vi "InitialPulseDelta6221_ver2.0.vi"(1 "Keithley6221 Compliance (V)":dbl=10.0, 2 "NV2182A range (V)":dbl=10.0, 4 "# of PLC":i16=10, 5 "Unit":string(combo)="V", 6 "Pluse Width  In (s)":dbl, 7 "Delay Time (s)":dbl, 8 "error in (no error)":errorcluster, 9 "Low Level In (A)":dbl, 10 "High Level In (A)":dbl, 11 "VISA Refnum in":refnum<visa-resource-name>) -> (0 "error out":errorcluster, 3 "VISA Refnum out":refnum<visa-resource-name>)   [LabVIEW 2012]
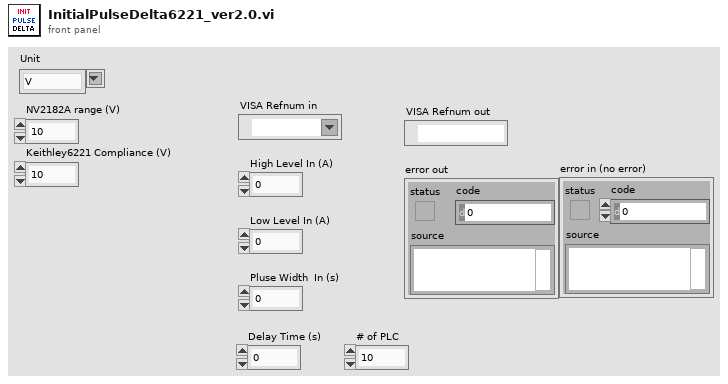
[diagram p1: front panel]
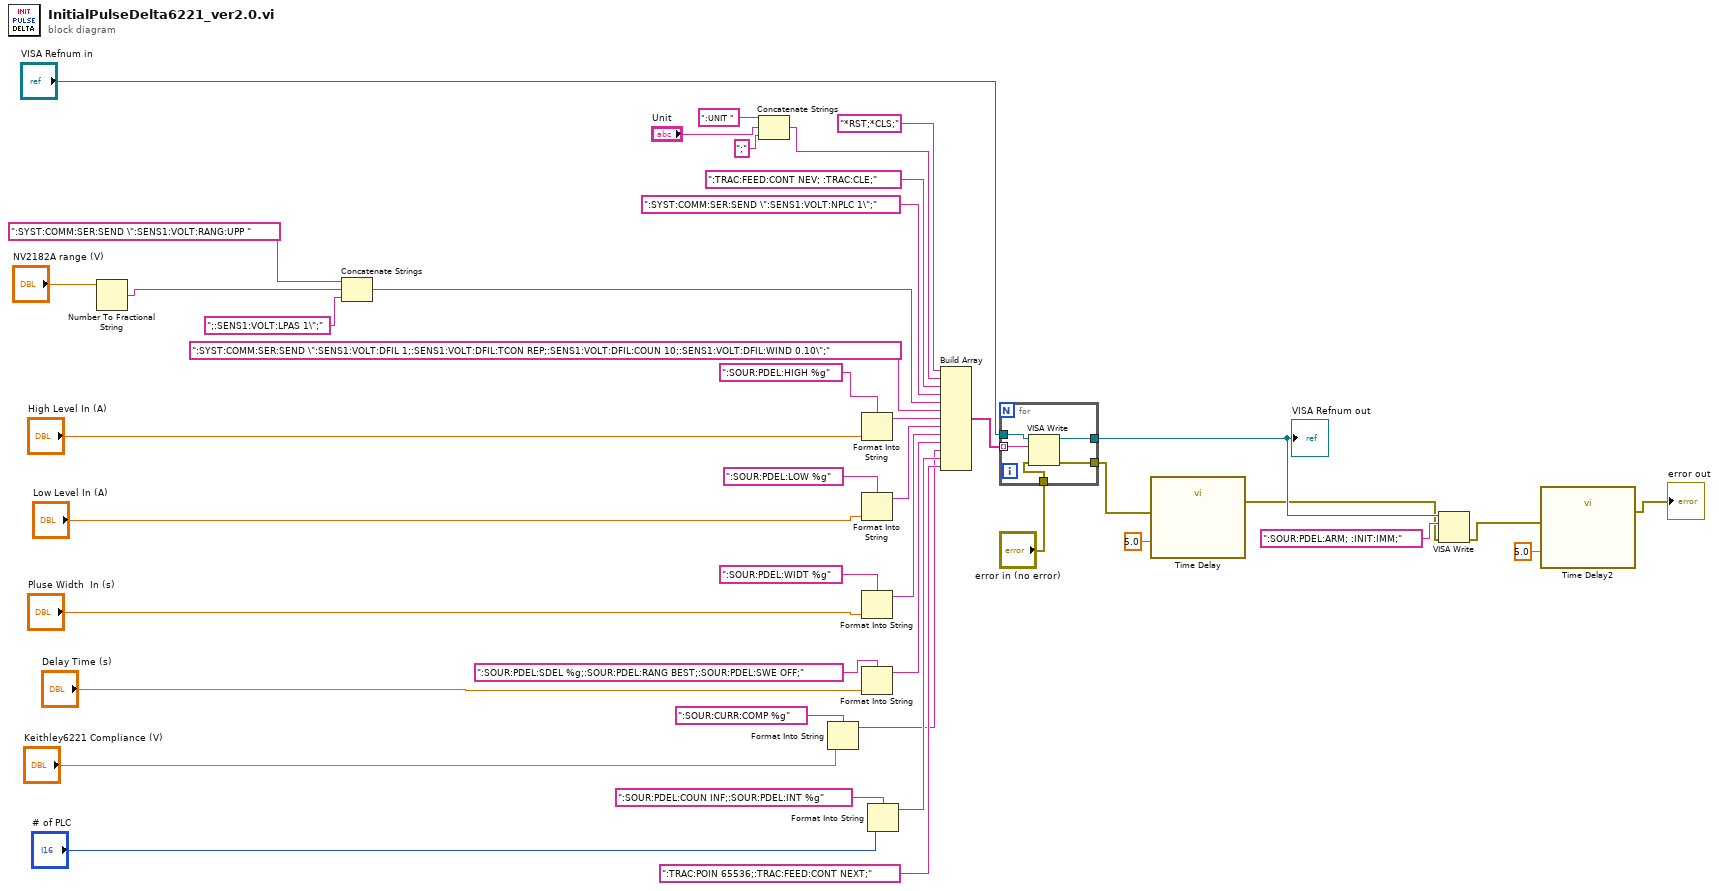
[diagram p0: block diagram]
diagram:
  n1 = Number To Fractional String(number="NV2182A range (V)") -> (F-format string=w3:string)  [unwired: 3 in]
  n2 = Concatenate Strings(":SYST:COMM:SER:SEND \":SENS1:VOLT:RANG:UPP " ("format string"), w3, ";:SENS1:VOLT:LPAS 1\";" ("format string")) -> (w1:string)
  n3 = Concatenate Strings(":UNIT " ("write buffer"), "Unit", ";" ("string")) -> (w9:string)
  n4 = Format Into String(format string=":SOUR:CURR:COMP %g", "Keithley6221 Compliance (V)") -> (resulting string=w6:string)  [unwired: 2 in, 1 out]
  n5 = Format Into String(format string=":SOUR:PDEL:HIGH %g", "High Level In (A)") -> (resulting string=w33:string)  [unwired: 2 in, 1 out]
  n6 = Format Into String(format string=":SOUR:PDEL:LOW %g", "Low Level In (A)") -> (resulting string=w32:string)  [unwired: 2 in, 1 out]
  n7 = Format Into String(format string=":SOUR:PDEL:WIDT %g", "Pluse Width  In (s)") -> (resulting string=w31:string)  [unwired: 2 in, 1 out]
  n8 = Format Into String(format string=":SOUR:PDEL:SDEL %g;:SOUR:PDEL:RANG BEST;:SOUR:PDEL:SWE OFF;", "Delay Time (s)") -> (resulting string=w42:string)  [unwired: 2 in, 1 out]
  n9 = Format Into String(format string=":SOUR:PDEL:COUN INF;:SOUR:PDEL:INT %g", "# of PLC") -> (resulting string=w22:string)  [unwired: 2 in, 1 out]
  n10 = Build Array("*RST;*CLS;" ("write buffer"), w9, ":TRAC:FEED:CONT NEV; :TRAC:CLE;" ("format string"), ":SYST:COMM:SER:SEND \":SENS1:VOLT:NPLC 1\";", w1, ":SYST:COMM:SER:SEND \":SENS1:VOLT:DFIL 1;:SENS1:VOLT:DFIL:TCON REP;:SENS1:VOLT:DFIL:COUN 10;:SENS1:VOLT:DFIL:WIND 0.10\";", w33, w32, w31, w42, w6, w22, ":TRAC:POIN 65536;:TRAC:FEED:CONT NEXT;" ("format string")) -> (w30:string[])
  n11 = for {
    tunnel: w30 -> [w48] mode=indexing
    tunnel: "VISA Refnum in" -> [w47]
    tunnel: [w46] -> w16
    tunnel: [w45] -> w20
    tunnel: "error in (no error)" -> [w44]
    n12 = VISA Write(VISA resource name=w47, write buffer=w48, error in (no error)=w44) -> (VISA resource name out=w46:refnum<visa-resource-name>, error out=w45:errorcluster)  [unwired: 1 out]
  }
  "VISA Refnum out" <- w16
  n13 = call "Time Delay"("error in (no error)"=w20, "Delay Time (s)"=5.0) -> ("error out"=w15:errorcluster)  [unwired: 9 in]
  n14 = VISA Write(VISA resource name=w16, write buffer=":SOUR:PDEL:ARM; :INIT:IMM;" ("format string"), error in (no error)=w15) -> (error out=w14:errorcluster)  [unwired: 2 out]
  n15 = call "Time Delay2"("error in (no error)"=w14, "Delay Time (s)"=5.0) -> ("error out"=→"error out":errorcluster)  [unwired: 9 in]
